vi "getRunnungMachine.vi"(10 "rc_no":string) -> (0 "error out":errorcluster, 3 "machine":string)   [LabVIEW 2012]
uses:
  <vilib>/addons/database/Connection.llb/DB Tools Open Connec (Path).vi
  <vilib>/addons/database/_DB Variant To Data/Database Variant To Data.xnode
  <vilib>/addons/database/NI_Database_API.lvlib
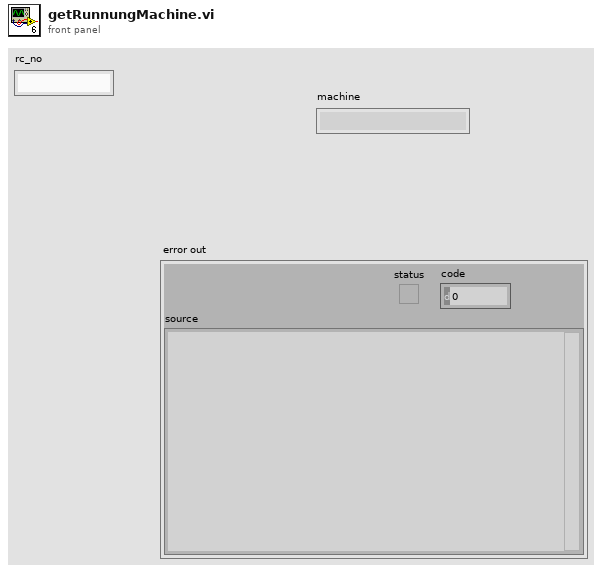
[diagram p1: front panel]
types:
  T1 = typedef "NI_Database_API.lvlib/Conn ObjectReference.ctl" = refnum<k1>
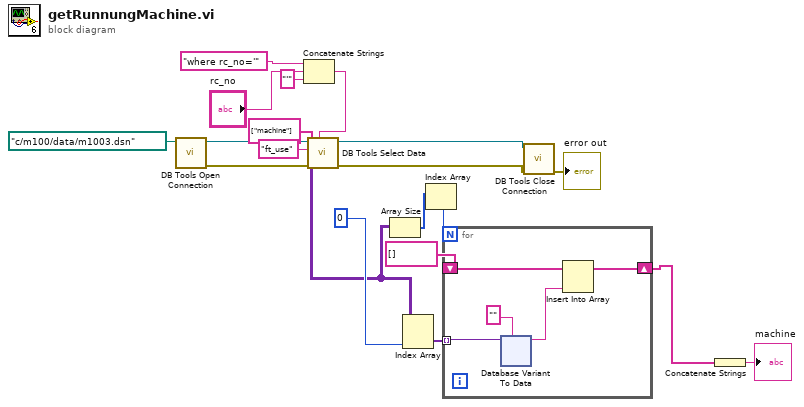
[diagram p0: block diagram]
diagram:
  n1 = call-poly <vilib>:"DB Tools Open Connection.vi"("connection information"=path "c:/m100/data/m1003.dsn") -> ("error out"=w17:errorcluster, "connection reference"=w18:T1)  [unwired: 7 in]
  n2 = Concatenate Strings("where rc_no='" ("condition"), "rc_no", "'" ("string")) -> (w9:string)
  n3 = call <vilib>:"DB Tools Select Data.vi"("condition"=w9, "error in (no error)"=w17, "columns"=string[] ["machine"], "table"="ft_use", "connection reference"=w18) -> ("error out"=w15:errorcluster, "data"=w6:variant[][], "connection reference out"=w16:T1)  [unwired: 1 in]
  n4 = Array Size(array=w6) -> (size(s)=w5:i32[])
  n5 = Index Array(array=w6, index (col)=0 ("disabled index (col)")) -> (element=w7:variant[])  [unwired: 1 in]
  n6 = Index Array(array=w5) -> (element=w4:i32)  [unwired: 1 in]
  n7 = for {
    N: w4 -> [_]
    tunnel: w7 -> [w25] mode=indexing
    shift-right: [w22] -> w2
    shift-left: string[] [] ("Array") -> [w21]
    n8 = xnode "Database Variant To Data"("database variant"=w25, "type"="") -> ("data"=w23:string)  [unwired: 1 in, 1 out]
    n9 = Insert Into Array(array=w21, new element=w23) -> (w22:string[])  [unwired: 1 in]
  }
  n10 = call <vilib>:"DB Tools Close Connection.vi"("error in (no error)"=w15, "connection reference"=w16) -> ("error out"=→"error out":errorcluster)  [unwired: 5 in]
  n11 = Concatenate Strings(w2) -> (→"machine":string)
